vi "Error Query.vi"(8 "error in (no error)":errorcluster, 11 "VISA resource name":refnum<visa-resource-name>) -> (0 "error out":errorcluster, 1 "Error Message":string, 2 "Error Code":i32[](array[numeric]), 3 "VISA resource name out":refnum<visa-resource-name>)   [LabVIEW 2018, in "Keithley 2600 Series.lvlib"]
doc: "Queries the instrument for any errors in the instrument's error queue. It will continue to read errors until all errors have been read from the instrument. Any errors will be returned in the <B>error out</B> control.\n\n<B>Note:</B>\nThis VI is called automatically by most driver VIs so it is not usually necessary to call this in an application.\n\n<b>Functions and Attributes Used</b>\nerrorqueue.next()"
uses:
  Keithley 2600 Series.lvlib
panel:
  # "(c) 2008 Keithley Instruments, Inc.  ALL RIGHTS RESERVED."
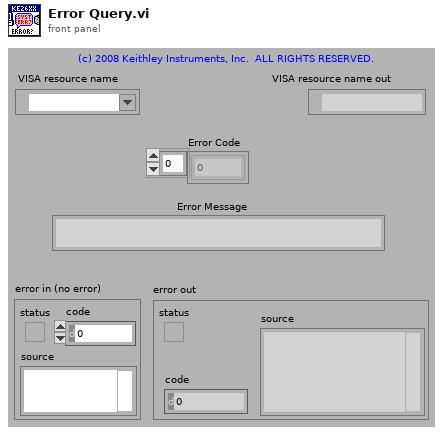
[diagram p1: front panel]
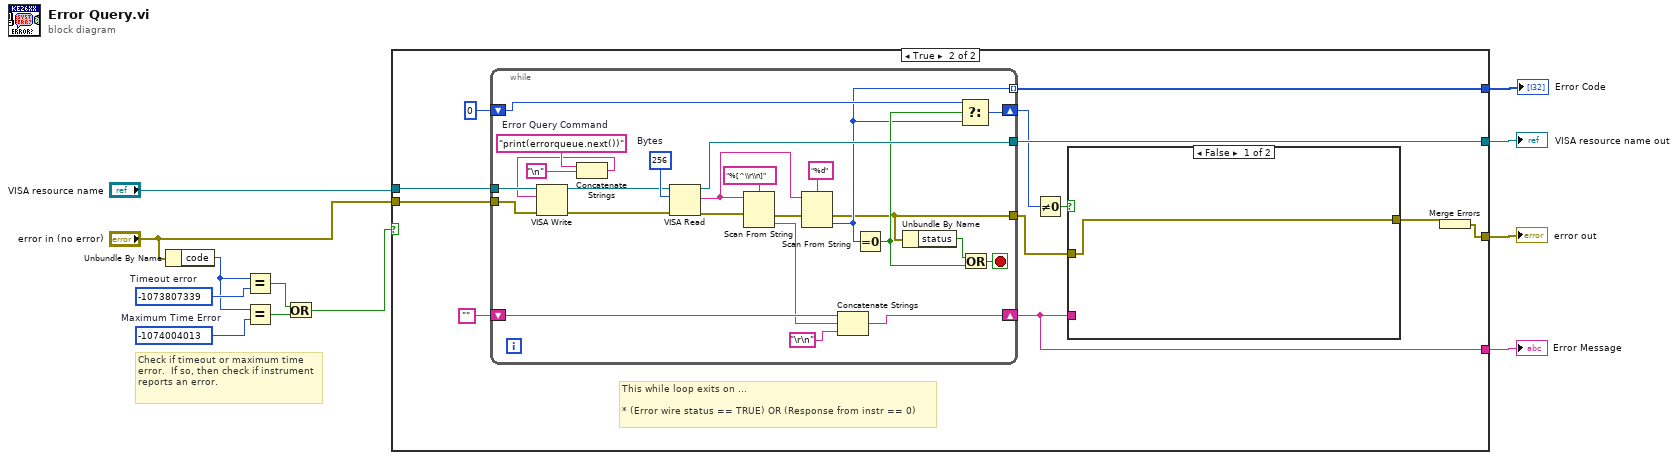
[diagram p0: block diagram]
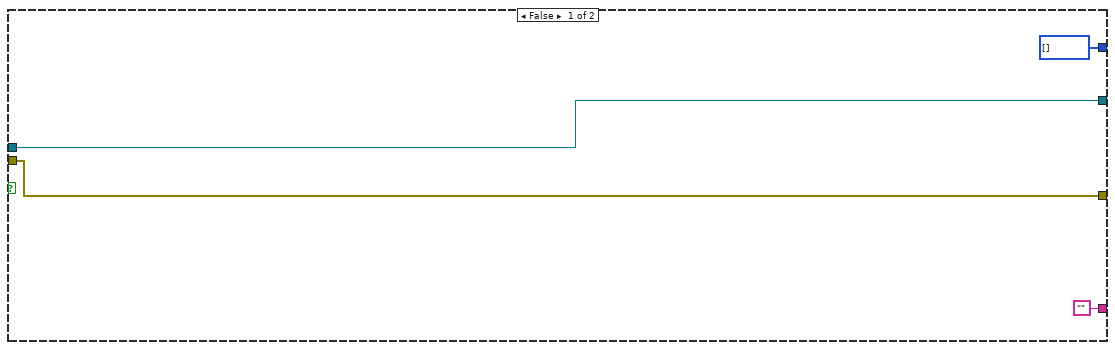
[diagram p2: hidden frame]
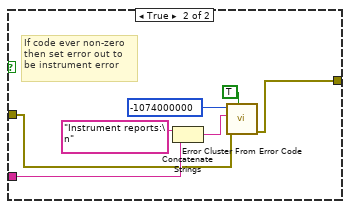
[diagram p3: hidden frame]
diagram:
  w6 = -1074004013  # Maximum Time Error
  w8 = -1073807339  # Timeout error
  # "Check if timeout or maximum time error.  If so, then check if instrument reports an error."
  n1 = Unbundle By Name("error in (no error)") -> ("code"=w7:i32)
  n2 = Equal?(x=w7, y=w8) -> (x = y?=w4:bool)
  n3 = Equal?(x=w7, y=w6) -> (x = y?=w5:bool)
  n4 = Or(x=w4, y=w5) -> (x .or. y?=w3:bool)
  n5 = case shown="True" w3 {
    tunnel: [w16 w28] -> w12
    tunnel: "VISA resource name" -> [w16 w27]
    tunnel: [w13 w25] -> w11
    tunnel: ["" w20] -> w10
    tunnel: [i32[] [] w19] -> w9
    tunnel: "error in (no error)" -> [w13 w18]
    frame False {
    }
    frame True {
      # "This while loop exits on ...\n\n* (Error wire status == TRUE) OR (Response from instr == 0)"
      n6 = while {
        tunnel: [w61] -> w28
        tunnel: w27 -> [w60]
        shift-right: [w51] -> w20
        shift-left: "" -> [w54]
        shift-right: [w49] -> w21
        shift-left: 0 -> [w50]
        tunnel: [w44] -> w19 mode=indexing
        tunnel: w18 -> [w40]
        tunnel: [w39] -> w17
        stop <- w57 stop-if-true
        w59 = u32 256  # Bytes
        w43 = "print(errorqueue.next())"  # Error Query Command
        n7 = Concatenate Strings(w43, "\n") -> (w41:string)
        n8 = VISA Write(VISA resource name=w60, write buffer=w41, error in (no error)=w40) -> (VISA resource name out=w37:refnum<visa-resource-name>, error out=w38:errorcluster)  [unwired: 1 out]
        n9 = VISA Read(VISA resource name=w37, byte count=w59, error in (no error)=w38) -> (VISA resource name out=w61:refnum<visa-resource-name>, read buffer=w55:string, error out=w48:errorcluster)  [unwired: 1 out]
        n10 = Scan From String(format string="%[^\\r\\n]", input string=w55, error in=w48) -> (error out=w47:errorcluster, output 1=w52:string)  [unwired: 1 in, 3 out]
        n11 = Scan From String(format string="%d", input string=w55, error in=w47) -> (error out=w39:errorcluster, output 1=w44:i32)  [unwired: 1 in, 3 out]
        n12 = Concatenate Strings(w54, w52, "\r\n") -> (w51:string)
        n13 = Equal To 0?(x=w44) -> (x = 0?=w45:bool)
        n14 = Unbundle By Name(w39) -> ("status"=w46:bool)
        n15 = Select(t=w50, s=w45, f=w44) -> (s? t:f=w49:i32)
        n16 = Or(x=w46, y=w45) -> (x .or. y?=w57:bool)
      }
      n17 = Not Equal To 0?(x=w21) -> (x != 0?=w23:bool)
      n18 = case shown="False" w23 {
        tunnel: w20 -> [_ w35]
        tunnel: [w29 w31] -> w22
        tunnel: w17 -> [w29 w30]
        frame False {
        }
        frame True {
          # "If code ever non-zero\nthen set error out to\nbe instrument error"
          n19 = Concatenate Strings("Instrument reports:\n" ("Source"), w35) -> (w32:string)
          n20 = call "Error Cluster From Error Code.vi"("show call chain? (False)"=TRUE, "error in (no error)"=w30, "error message (\"\")"=w32, "error code (0)"=-1074000000 ("Code")) -> ("error out"=w31:errorcluster)  [unwired: 5 out]
        }
      }
      n21 = Merge Errors(w22) -> (w25:errorcluster)
    }
  }
  "VISA resource name out" <- w12
  "error out" <- w11
  "Error Message" <- w10
  "Error Code" <- w9
